vi "FestoCPX.Station.ProdPresent.Check.vi"(6 "Stab Counter (0)":i32, 8 "error in":errorcluster) -> (0 "error out":errorcluster, 1 "table empty (all out)":bool, 2 "Prod Present":T1, 3 "#products in the machine":i32, 4 "Final Stab time [ms]":u32, 5 "Final amount":i32)   [LabVIEW 2016]
uses:
  FestoCPX.Station.ProdPresent.ctl
  FestoCPX.DI.Signal.ctl
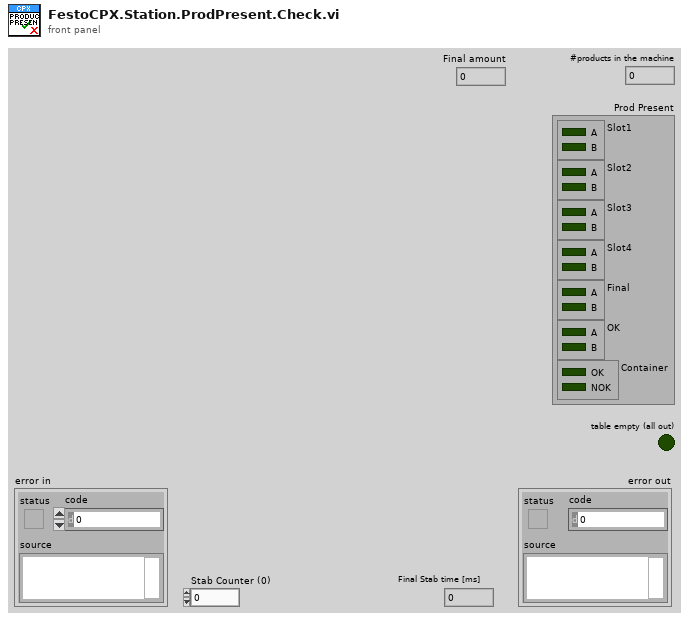
[diagram p1: front panel]
types:
  T1 = typedef "FestoCPX.Station.ProdPresent.ctl" = cluster{"Slot1":cluster{"A":bool, "B":bool}, "Slot2":cluster{"A":bool, "B":bool}, "Slot3":cluster{"A":bool, "B":bool}, "Slot4":cluster{"A":bool, "B":bool}, "Final":cluster{"A":bool, "B":bool}, "OK":cluster{"A":bool, "B":bool}, "Container":cluster{"OK":bool, "NOK":bool}}
  T2 = typedef "FestoCPX.DI.Signal.ctl" = enum16{"S.C. Emergency Stop", "S.C. Side Door Close", "S.C. Front Door Close", "S.C. Front Door Secured", "Button Start", "Button Stop", "Button Control", "Product Move Home", "Product Move Work", "Table Position", "Table Lock", "Product Lift A Home", "Product Lift B Home", "Product Arm OK", "Product Arm NOK", "Product Arm Work", "Revolver ID 1", "Revolver ID 2", "Revolver ID 3", "Revolver ID 4", "Revolver ID 5", "Air Pressure Inside", "Air Pressure Inlet", "Product Slot 1 A Present", "Product Slot 1 B Present", "Product Slot 2 A Present", "Product Slot 2 B Present", "Product Slot 3 A Present", "Product Slot 3 B Present", "Product Slot 4 A Present", "Product Slot 4 B Present", "Product Final A Present", "Product Final B Present", "Product Output A Present", "Product Output B Present", "Product Container OK Present", "Product Container NOK Present", "Fork ID 1", "Fork ID 2"}
  T3 = cluster{cluster{"Run":bool, "Run":bool}, cluster{"Run":bool, "Run":bool}, cluster{"Run":bool, "Run":bool}, cluster{"Run":bool, "Run":bool}, cluster{"Run":bool, "Run":bool}, cluster{"Run":bool, "Run":bool}, cluster{"Run":bool, "Run":bool}}
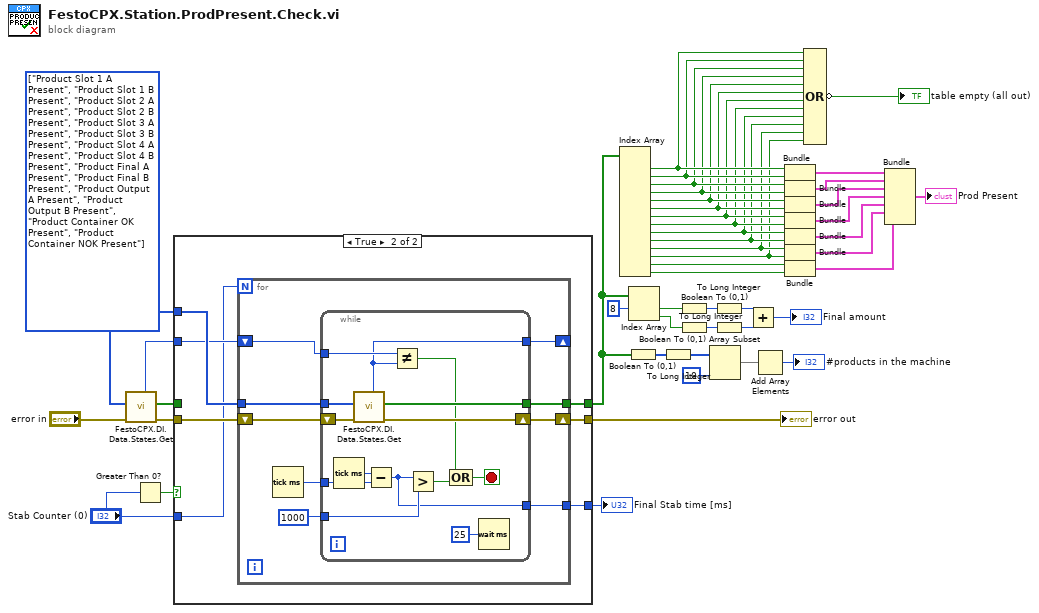
[diagram p0: block diagram]
diagram:
  w6 = T2[] [enum."Product Slot 1 A Present", enum."Product Slot 1 B Present", enum."Product Slot 2 A Present", enum."Product Slot 2 B Present", enum."Product Slot 3 A Present", enum."Product Slot 3 B Present", enum."Product Slot 4 A Present", enum."Product Slot 4 B Present", enum."Product Final A Present", enum."Product Final B Present", enum."Product Output A Present", enum."Product Output B Present", enum."Product Container OK Present", enum."Product Container NOK Present"] items=["S.C. Emergency Stop", "S.C. Side Door Close", "S.C. Front Door Close", "S.C. Front Door Secured", "Button Start", "Button Stop", "Button Control", "Product Move Home", "Product Move Work", "Table Position", "Table Lock", "Product Lift A Home", "Product Lift B Home", "Product Arm OK", "Product Arm NOK", "Product Arm Work", "Revolver ID 1", "Revolver ID 2", "Revolver ID 3", "Revolver ID 4", "Revolver ID 5", "Air Pressure Inside", "Air Pressure Inlet", "Product Slot 1 A Present", "Product Slot 1 B Present", "Product Slot 2 A Present", "Product Slot 2 B Present", "Product Slot 3 A Present", "Product Slot 3 B Present", "Product Slot 4 A Present", "Product Slot 4 B Present", "Product Final A Present", "Product Final B Present", "Product Output A Present", "Product Output B Present", "Product Container OK Present", "Product Container NOK Present", "Fork ID 1", "Fork ID 2"] ("CPX.DI")
  n1 = call "FestoCPX.DI.Data.States.Get.vi"("error in (no error)"="error in", "CPX.DI"=w6) -> ("error out"=w7:errorcluster, "State OR"=w2:bool[], "FrameCounter"=w5:i32)  [unwired: 5 in, 2 out]
  n2 = Greater Than 0?(x="Stab Counter (0)") -> (x > 0?=w3:bool)
  n3 = case shown="True" w3 {
    tunnel: [w47 w55] -> w46
    tunnel: [w48 w54] -> w9
    tunnel: w7 -> [w47 w53]
    tunnel: w6 -> [_ w52]
    tunnel: w5 -> [_ w51]
    tunnel: "Stab Counter (0)" -> [_ w49]
    tunnel: w2 -> [w48 _]
    tunnel: [_ w50] -> w1
    frame False {
    }
    frame True {
      n4 = for {
        N: w49 -> [_]
        tunnel: [w63] -> w54
        tunnel: w52 -> [w60]
        tunnel: [w58] -> w50
        shift-right: [w64] -> w55
        shift-left: w53 -> [w61]
        shift-right: [w56] -> _
        shift-left: w51 -> [w59]
        n5 = Tick Count (ms)() -> (millisecond timer value=w62:u32)
        n6 = while {
          tunnel: w60 -> [w76]
          tunnel: [w75] -> w63
          shift-right: [w78] -> w64
          shift-left: w61 -> [w77]
          tunnel: w62 -> [w73]
          tunnel: w59 -> [w72]
          tunnel: u32 1000 ("Max Stab time [ms] (0)") -> [w68]
          tunnel: [w67] -> w58
          tunnel: [w65] -> w56
          stop <- w70 stop-if-true
          n7 = Tick Count (ms)() -> (millisecond timer value=w74:u32)
          n8 = call "FestoCPX.DI.Data.States.Get.vi"("error in (no error)"=w77, "CPX.DI"=w76) -> ("error out"=w78:errorcluster, "State OR"=w75:bool[], "FrameCounter"=w65:i32)  [unwired: 5 in, 2 out]
          n9 = Subtract(x=w74, y=w73) -> (x-y=w67:u32)
          n10 = Not Equal?(x=w72, y=w65) -> (x != y?=w66:bool)
          n11 = Greater?(x=w67, y=w68) -> (0:w71:bool)
          n12 = Compound Arithmetic op=OR(w66, w71) -> (w70:bool)
          n13 = Wait (ms)(milliseconds to wait=u32 25) -> ()  [unwired: 1 out]
        }
      }
    }
  }
  "error out" <- w46
  "Final Stab time [ms]" <- w1
  n14 = Index Array(array=w9) -> (element #1=w45:bool, element #2=w44:bool, element #3=w39:bool, element #4=w38:bool, element #5=w36:bool, element #6=w35:bool, element #7=w34:bool, element #8=w33:bool, element #9=w26:bool, element #10=w25:bool, element #11=w24:bool, element #12=w23:bool, element #13=w29:bool, element #14=w28:bool)  [unwired: 14 in]
  n15 = Boolean To (0,1)(Boolean=w9) -> (0, 1=w22:i16[])
  n16 = Index Array(array=w9, index #1=8 ("index")) -> (element #1=w15:bool, element #2=w13:bool)  [unwired: 1 in]
  n17 = To Long Integer(number=w22) -> (32bit integer=w18:i32[])
  n18 = Boolean To (0,1)(Boolean=w15) -> (0, 1=w16:i16)
  n19 = Boolean To (0,1)(Boolean=w13) -> (0, 1=w14:i16)
  n20 = Array Subset(array=w18, length=10) -> (w20:i32[])  [unwired: 1 in]
  n21 = To Long Integer(number=w16) -> (32bit integer=w12:i32)
  n22 = To Long Integer(number=w14) -> (32bit integer=w11:i32)
  n23 = Add(x=w12, y=w11) -> (x+y=→"Final amount":i32)
  n24 = Add Array Elements(numeric array=w20) -> (sum=→"#products in the machine":i32)
  n25 = Bundle("Run"=w45, "Run"=w44) -> (w43:cluster{"Run":bool, "Run":bool})  [unwired: 1 in]
  n26 = Bundle("Run"=w39, "Run"=w38) -> (w42:cluster{"Run":bool, "Run":bool})  [unwired: 1 in]
  n27 = Bundle("Run"=w36, "Run"=w35) -> (w41:cluster{"Run":bool, "Run":bool})  [unwired: 1 in]
  n28 = Bundle("Run"=w34, "Run"=w33) -> (w40:cluster{"Run":bool, "Run":bool})  [unwired: 1 in]
  n29 = Bundle("Run"=w26, "Run"=w25) -> (w31:cluster{"Run":bool, "Run":bool})  [unwired: 1 in]
  n30 = Bundle("Run"=w24, "Run"=w23) -> (w30:cluster{"Run":bool, "Run":bool})  [unwired: 1 in]
  n31 = Bundle("Run"=w29, "Run"=w28) -> (w27:cluster{"Run":bool, "Run":bool})  [unwired: 1 in]
  n32 = Compound Arithmetic op=OR(w45, w44, w39, w38, w36, w35, w34, w33, w26, w25, w24, w23) -> (invert →"table empty (all out)":bool)
  n33 = Bundle(w43, w42, w41, w40, w31, w30, w27) -> (→"Prod Present":T3)  [unwired: 1 in]
